vi "Read System Circular Buffers.vi"(8 "error in (no error)":errorcluster, 11 "Root Actor in":refnum<class "Root Actor.lvclass">) -> (0 "error out":errorcluster, 2 "System Circular Buffers":refnum<class "Circular Buffer.lvclass">[](array[class]), 3 "Root Actor out":refnum<class "Root Actor.lvclass">)   [LabVIEW 2019, in "Root Actor.lvclass"]
uses:
  Root Actor.lvclass
  Circular Buffer/Circular Buffer.lvclass
  Root Actor.lvclass/Root Actor.ctl
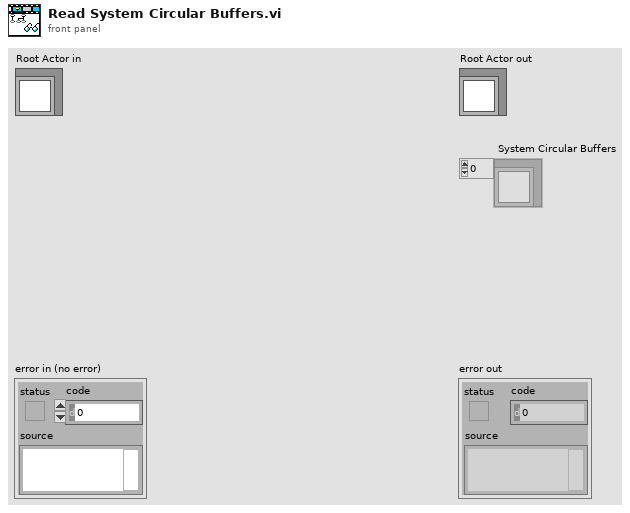
[diagram p1: front panel]
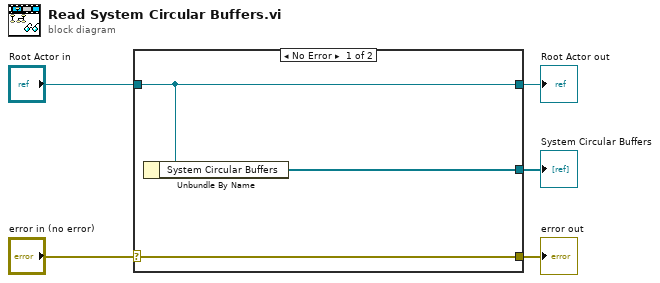
[diagram p0: block diagram]
diagram:
  n1 = case shown="No Error" "error in (no error)" {
    selector: "error in (no error)" -> [w8 w9]
    tunnel: [w8 w9] -> w4
    tunnel: [w7 w10] -> w2
    tunnel: "Root Actor in" -> [w7 w10]
    tunnel: [w6 _] -> w1
    frame No Error {
      n2 = Unbundle By Name(w7) -> ("System Circular Buffers"=w6:refnum<class "Circular Buffer.lvclass">[])
    }
    frame Error {
    }
  }
  "error out" <- w4
  "Root Actor out" <- w2
  "System Circular Buffers" <- w1
